vi "APXTurboEPICS.vi"() -> ()   [LabVIEW 2015]
uses:
  <vilib>/Instr/_visa.llb/VISA Configure Serial Port (Instr).vi
  <userlib>/caLab/Private/Get_PV-1D.vi
  <userlib>/caLab/Private/Put_DBL_PV.vi
  <userlib>/caLab/Private/Put_DBL-1D_PV-1D.vi
panel:
  out "APX:GASTurbo_START":bool
  out "APX:GASTrubo_STOP":bool
  out "APX:GASTurboF":dbl caption="F_20/Hz"
  out "APX:GASTurboP":dbl caption="P_20/W"
  out "APX:GASTurboS:STR":string
  out "APX:GASTurboS":dbl
  out "SERIAL 5":string
  out "GASTurbo":refnum<visa-resource-name>="COM4"
  out "APX:HPCTurbo_START":bool
  out "APX:HPCTrubo_STOP":bool
  out "APX:HPCTurboF":dbl caption="F_20/Hz"
  out "APX:HPCTurboP":dbl caption="P_20/W"
  out "APX:HPCTurboS:STR":string
  out "APX:HPCTurboS":dbl
  out "SERIAL 4":string
  out "HPCTurbo":refnum<visa-resource-name>="COM4"
  out "SERIAL 3":string
  out "L2Turbo":refnum<visa-resource-name>="COM4"
  out "APX:L2Turbo_START":bool
  out "APX:L2Turbo_STOP":bool
  out "APX:L2TurboF":dbl caption="F_20/Hz"
  out "APX:L2TurboP":dbl caption="P_20/W"
  out "APX:L2TurboS:STR":string
  out "AP2:L2TruboS":dbl
  out "SERIAL 2":string
  out "AP2Turbo":refnum<visa-resource-name>="COM4"
  out "APX:AP2Turbo_START":bool
  out "APX:AP2Trubo_STOP":bool
  out "APX:AP2TurboF":dbl caption="F_20/Hz"
  out "APX:AP2TurboP":dbl caption="P_20/W"
  out "APX:AP2TurboS:STR":string
  out "APX:AP2TruboS":dbl
  out "APX:HEMTurboS":dbl
  out "APX:HEMTurbo_STOP":bool
  out "APX:HEMTurbo_START":bool
  out "HEMTurbo":refnum<visa-resource-name>="COM4"
  out "APX:HEMTurboF":dbl caption="F_20/Hz"
  out "APX:HEMTurboP":dbl caption="P_20/W"
  out "APX:HEMTurboS:STR":string
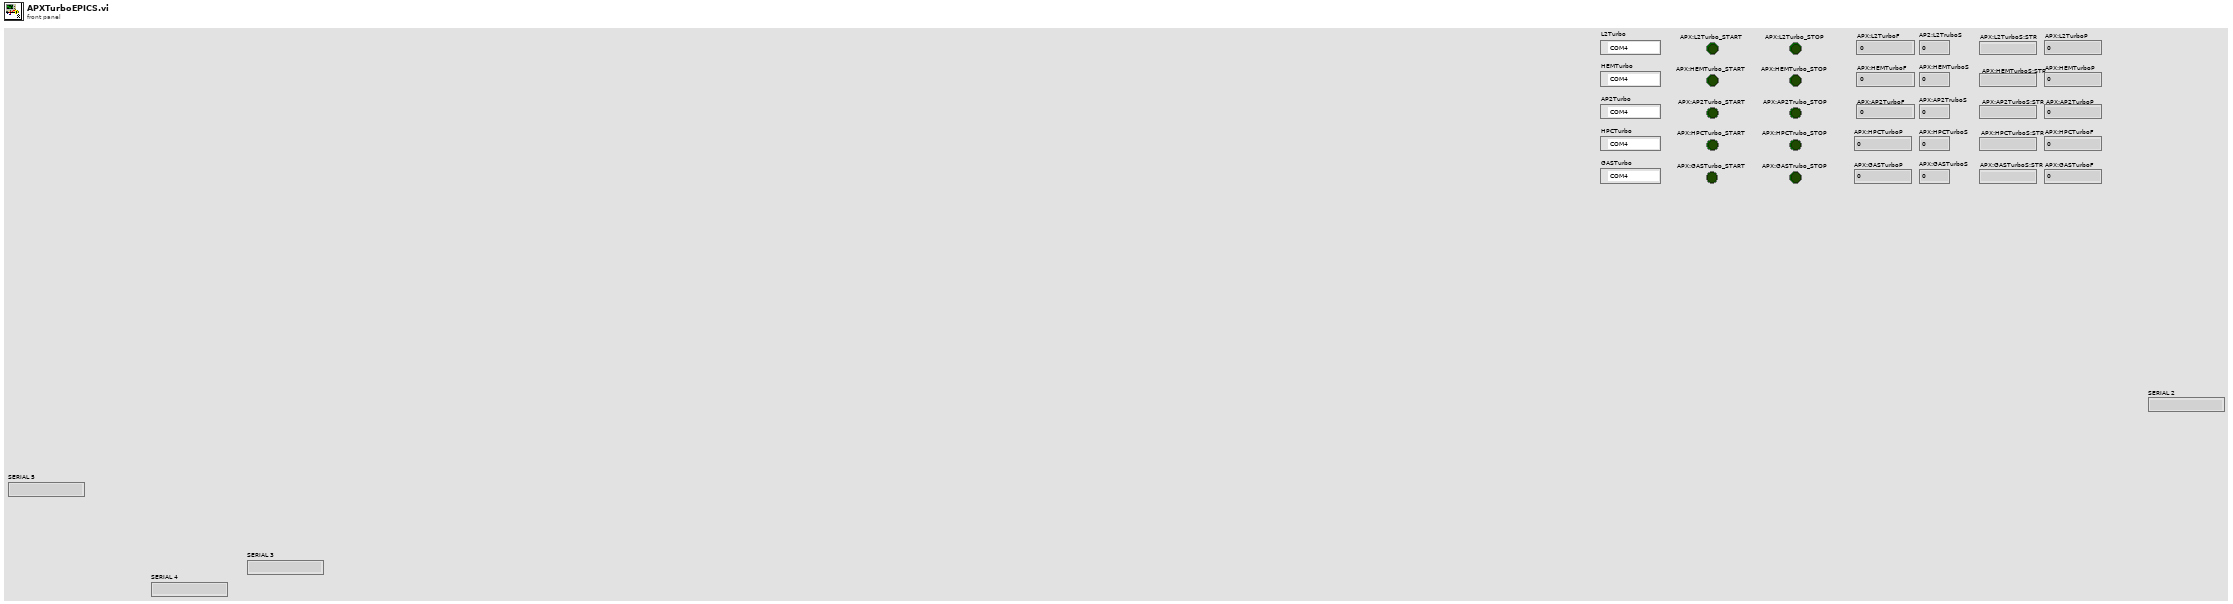
[diagram p1: front panel]
types:
  T1 = enum16{"START", "STOP", "REMOTE/SERIAL", "REMOTE", "SERIAL", "START/STOP", "PUMP STATUS", "Driving Frequency", "PUMP POWER", "PRESSURE"}
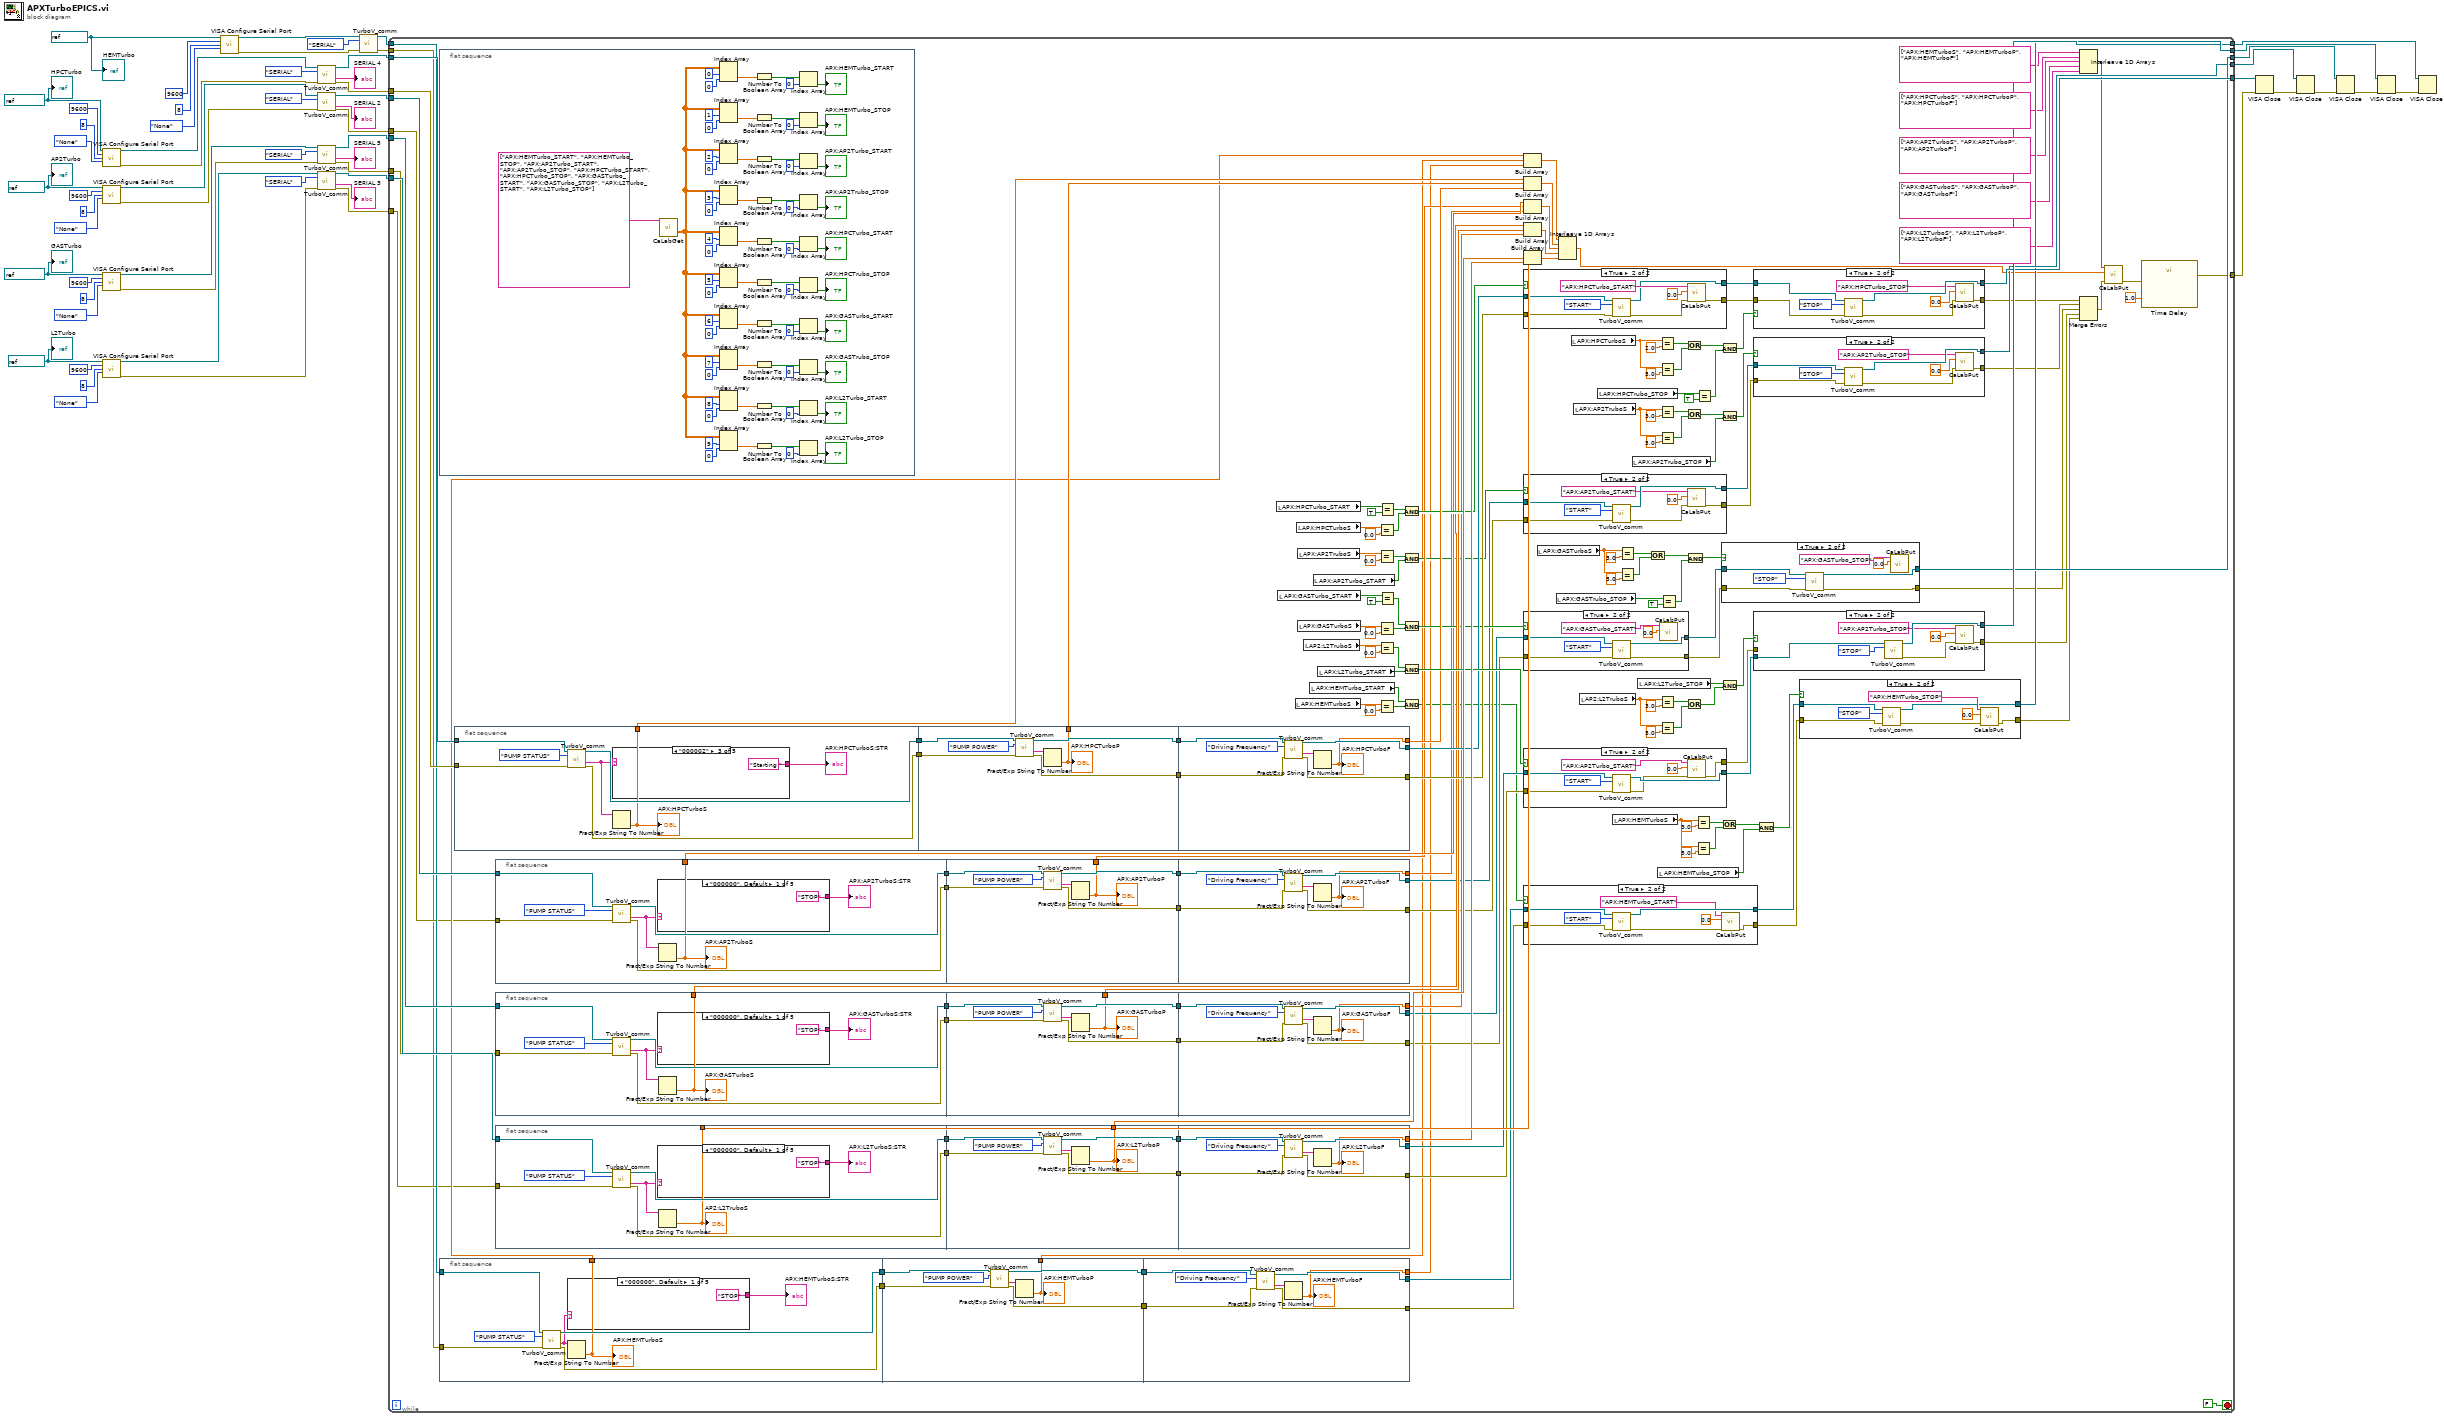
[diagram p0: block diagram]
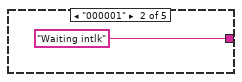
[diagram p2: hidden frame]
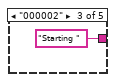
[diagram p3: hidden frame]
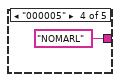
[diagram p4: hidden frame]
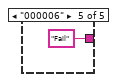
[diagram p5: hidden frame]
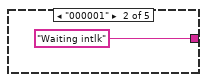
[diagram p8: hidden frame]
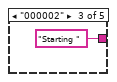
[diagram p9: hidden frame]
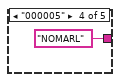
[diagram p10: hidden frame]
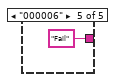
[diagram p11: hidden frame]
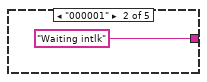
[diagram p14: hidden frame]
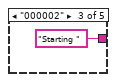
[diagram p15: hidden frame]
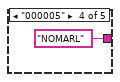
[diagram p16: hidden frame]
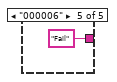
[diagram p17: hidden frame]
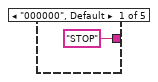
[diagram p20: hidden frame]
diagram:
  w18 = refnum<visa-resource-name> "COM25" ("VISA resource name")
  w33 = refnum<visa-resource-name> "COM26" ("VISA resource name")
  w44 = refnum<visa-resource-name> "COM4" ("VISA resource name")
  w52 = refnum<visa-resource-name> "COM6" ("VISA resource name")
  w59 = refnum<visa-resource-name> "COM5" ("VISA resource name")
  n1 = call-poly "VISA Configure Serial Port"("VISA resource name"=w18, "baud rate (9600)"=u32 9600, "data bits (8)"=u16 8, "parity (0:none)"=enum16{"None", "Odd", "Even", "Mark", "Space"}."None") -> ("VISA resource name out"=w23:refnum<visa-resource-name>, "error out"=w24:errorcluster)  [unwired: 10 in]
  n2 = call-poly "VISA Configure Serial Port"("VISA resource name"=w52, "baud rate (9600)"=u32 9600, "data bits (8)"=u16 8, "parity (0:none)"=enum16{"None", "Odd", "Even", "Mark", "Space"}."None") -> ("VISA resource name out"=w47:refnum<visa-resource-name>, "error out"=w46:errorcluster)  [unwired: 10 in]
  n3 = call-poly "VISA Configure Serial Port"("VISA resource name"=w33, "baud rate (9600)"=u32 9600, "data bits (8)"=u16 8, "parity (0:none)"=enum16{"None", "Odd", "Even", "Mark", "Space"}."None") -> ("VISA resource name out"=w28:refnum<visa-resource-name>, "error out"=w27:errorcluster)  [unwired: 10 in]
  n4 = call-poly "VISA Configure Serial Port"("VISA resource name"=w44, "baud rate (9600)"=u32 9600, "data bits (8)"=u16 8, "parity (0:none)"=enum16{"None", "Odd", "Even", "Mark", "Space"}."None") -> ("VISA resource name out"=w38:refnum<visa-resource-name>, "error out"=w36:errorcluster)  [unwired: 10 in]
  n5 = call-poly "VISA Configure Serial Port"("VISA resource name"=w59, "baud rate (9600)"=u32 9600, "data bits (8)"=u16 8, "parity (0:none)"=enum16{"None", "Odd", "Even", "Mark", "Space"}."None") -> ("VISA resource name out"=w54:refnum<visa-resource-name>, "error out"=w53:errorcluster)  [unwired: 10 in]
  n6 = call "TurboV_comm.vi"("VISA resource name"=w23, "Command"=T1."SERIAL", "error in (no error)"=w24) -> ("VISA resource name out"=w17:refnum<visa-resource-name>, "read buffer"=→"SERIAL 4":string, "error out"=w16:errorcluster)  [unwired: 10 in]
  n7 = call "TurboV_comm.vi"("VISA resource name"=w47, "Command"=T1."SERIAL", "error in (no error)"=w46) -> ("VISA resource name out"=w10:refnum<visa-resource-name>, "read buffer"=→"SERIAL 2":string, "error out"=w9:errorcluster)  [unwired: 10 in]
  n8 = call "TurboV_comm.vi"("VISA resource name"=w28, "Command"=T1."SERIAL", "error in (no error)"=w27) -> ("VISA resource name out"=w13:refnum<visa-resource-name>, "read buffer"=→"SERIAL 5":string, "error out"=w12:errorcluster)  [unwired: 10 in]
  n9 = call "TurboV_comm.vi"("VISA resource name"=w38, "Command"=T1."SERIAL", "error in (no error)"=w36) -> ("VISA resource name out"=w37:refnum<visa-resource-name>, "read buffer"=→"SERIAL 3":string, "error out"=w35:errorcluster)  [unwired: 10 in]
  n10 = call "TurboV_comm.vi"("VISA resource name"=w54, "Command"=T1."SERIAL", "error in (no error)"=w53) -> ("VISA resource name out"=w7:refnum<visa-resource-name>, "error out"=w6:errorcluster)  [unwired: 10 in, 1 out]
  n11 = while {
    tunnel: w37 -> [w224]
    tunnel: w35 -> [w82]
    tunnel: [w204] -> w40
    tunnel: w17 -> [w197]
    tunnel: w16 -> [w196]
    tunnel: [w167] -> w15
    tunnel: [w79] -> w14
    tunnel: w13 -> [w166]
    tunnel: w12 -> [w165]
    tunnel: [w164] -> w11
    tunnel: w10 -> [w135]
    tunnel: w9 -> [w83]
    tunnel: [w110] -> w8
    tunnel: w7 -> [w109]
    tunnel: w6 -> [w81]
    tunnel: [w80] -> w2
    stop <- FALSE stop-if-true
    n12 = flat-sequence {
      frame #0 {
        n13 = call-poly "CaLabGet.vi"("PV Names"=string[] ["APX:HEMTurbo_START", "APX:HEMTurbo_STOP", "APX:AP2Turbo_START", "APX:AP2Turbo_STOP", "APX:HPCTurbo_START", "APX:HPCTurbo_STOP", "APX:GASTurbo_START", "APX:GASTurbo_STOP", "APX:L2Turbo_START", "APX:L2Turbo_STOP"]) -> ("Value Array (number)"=w225:dbl[][])  [unwired: 8 in, 6 out]
        n14 = Index Array(array=w225, index (row)=0 ("disabled index (row)"), index (col)=0 ("index (row)")) -> (element=w233:dbl)
        n15 = Index Array(array=w225, index (row)=1 ("disabled index (row)"), index (col)=0 ("index (row)")) -> (element=w228:dbl)
        n16 = Index Array(array=w225, index (row)=2 ("disabled index (row)"), index (col)=0 ("index (row)")) -> (element=w246:dbl)
        n17 = Index Array(array=w225, index (row)=3 ("disabled index (row)"), index (col)=0 ("index (row)")) -> (element=w241:dbl)
        n18 = Index Array(array=w225, index (row)=4 ("disabled index (row)"), index (col)=0 ("index (row)")) -> (element=w270:dbl)
        n19 = Index Array(array=w225, index (row)=5 ("disabled index (row)"), index (col)=0 ("index (row)")) -> (element=w264:dbl)
        n20 = Index Array(array=w225, index (row)=6 ("disabled index (row)"), index (col)=0 ("index (row)")) -> (element=w258:dbl)
        n21 = Index Array(array=w225, index (row)=7 ("disabled index (row)"), index (col)=0 ("index (row)")) -> (element=w253:dbl)
        n22 = Index Array(array=w225, index (row)=8 ("disabled index (row)"), index (col)=0 ("index (row)")) -> (element=w282:dbl)
        n23 = Index Array(array=w225, index (row)=9 ("disabled index (row)"), index (col)=0 ("index (row)")) -> (element=w277:dbl)
        n24 = Number To Boolean Array(number=w233) -> (Boolean array=w235:bool[])
        n25 = Number To Boolean Array(number=w228) -> (Boolean array=w230:bool[])
        n26 = Number To Boolean Array(number=w246) -> (Boolean array=w248:bool[])
        n27 = Number To Boolean Array(number=w241) -> (Boolean array=w243:bool[])
        n28 = Number To Boolean Array(number=w270) -> (Boolean array=w272:bool[])
        n29 = Number To Boolean Array(number=w264) -> (Boolean array=w266:bool[])
        n30 = Number To Boolean Array(number=w258) -> (Boolean array=w260:bool[])
        n31 = Number To Boolean Array(number=w253) -> (Boolean array=w255:bool[])
        n32 = Number To Boolean Array(number=w282) -> (Boolean array=w284:bool[])
        n33 = Number To Boolean Array(number=w277) -> (Boolean array=w279:bool[])
        n34 = Index Array(array=w235, index=0) -> (element=→"APX:HEMTurbo_START":bool)
        n35 = Index Array(array=w230, index=0) -> (element=→"APX:HEMTurbo_STOP":bool)
        n36 = Index Array(array=w248, index=0) -> (element=→"APX:AP2Turbo_START":bool)
        n37 = Index Array(array=w243, index=0) -> (element=→"APX:AP2Trubo_STOP":bool)
        n38 = Index Array(array=w272, index=0) -> (element=→"APX:HPCTurbo_START":bool)
        n39 = Index Array(array=w266, index=0) -> (element=→"APX:HPCTrubo_STOP":bool)
        n40 = Index Array(array=w260, index=0) -> (element=→"APX:GASTurbo_START":bool)
        n41 = Index Array(array=w255, index=0) -> (element=→"APX:GASTrubo_STOP":bool)
        n42 = Index Array(array=w284, index=0) -> (element=→"APX:L2Turbo_START":bool)
        n43 = Index Array(array=w279, index=0) -> (element=→"APX:L2Turbo_STOP":bool)
      }
    }
    n44 = flat-sequence {
      tunnel: w109 -> [w294]
      tunnel: w81 -> [w293]
      tunnel: [w292] -> w107
      tunnel: [w291] -> w106
      tunnel: [w287] -> w103
      tunnel: w107 -> [w305]
      tunnel: w106 -> [w302]
      tunnel: [w304] -> w105
      tunnel: [w303] -> w104
      tunnel: [w300] -> w102
      tunnel: w105 -> [w313]
      tunnel: w104 -> [w312]
      tunnel: [w309] -> w92
      tunnel: [w308] -> w108
      tunnel: [w307] -> w101
      frame #0 {
        n45 = call "TurboV_comm.vi"("VISA resource name"=w294, "Command"=T1."PUMP STATUS", "error in (no error)"=w293) -> ("VISA resource name out"=w292:refnum<visa-resource-name>, "read buffer"=w288:string, "error out"=w291:errorcluster)  [unwired: 10 in]
        n46 = case shown="\"000000\", Default" w288 {
          tunnel: ["STOP" "Waiting intlk" "Starting " "NOMARL" "Fail"] -> w289
          frame "000000", Default {
          }
          frame "000001" {
          }
          frame "000002" {
          }
          frame "000005" {
          }
          frame "000006" {
          }
        }
        "APX:HEMTurboS:STR" <- w289
        n47 = Fract/Exp String To Number(string=w288) -> (number=w287:dbl)  [unwired: 3 in, 1 out]
        "APX:HEMTurboS" <- w287
      }
      frame #1 {
        n48 = call "TurboV_comm.vi"("VISA resource name"=w305, "Command"=T1."PUMP POWER", "error in (no error)"=w302) -> ("VISA resource name out"=w304:refnum<visa-resource-name>, "read buffer"=w301:string, "error out"=w303:errorcluster)  [unwired: 10 in]
        n49 = Fract/Exp String To Number(string=w301) -> (number=w300:dbl)  [unwired: 3 in, 1 out]
        "APX:HEMTurboP" <- w300
      }
      frame #2 {
        n50 = call "TurboV_comm.vi"("VISA resource name"=w313, "Command"=T1."Driving Frequency", "error in (no error)"=w312) -> ("VISA resource name out"=w308:refnum<visa-resource-name>, "read buffer"=w310:string, "error out"=w309:errorcluster)  [unwired: 10 in]
        n51 = Fract/Exp String To Number(string=w310) -> (number=w307:dbl)  [unwired: 3 in, 1 out]
        "APX:HEMTurboF" <- w307
      }
    }
    n52 = flat-sequence {
      tunnel: w197 -> [w433]
      tunnel: w196 -> [w432]
      tunnel: [w431] -> w195
      tunnel: [w430] -> w194
      tunnel: [w426] -> w191
      tunnel: w195 -> [w444]
      tunnel: w194 -> [w441]
      tunnel: [w443] -> w193
      tunnel: [w442] -> w192
      tunnel: [w439] -> w190
      tunnel: w193 -> [w452]
      tunnel: w192 -> [w451]
      tunnel: [w448] -> w179
      tunnel: [w447] -> w180
      tunnel: [w446] -> w189
      frame #0 {
        n53 = call "TurboV_comm.vi"("VISA resource name"=w433, "Command"=T1."PUMP STATUS", "error in (no error)"=w432) -> ("VISA resource name out"=w431:refnum<visa-resource-name>, "read buffer"=w427:string, "error out"=w430:errorcluster)  [unwired: 10 in]
        n54 = case shown="\"000002\"" w427 {
          tunnel: ["STOP" "Waiting intlk" "Starting " "NOMARL" "Fail"] -> w428
          frame "000000", Default {
          }
          frame "000001" {
          }
          frame "000002" {
          }
          frame "000005" {
          }
          frame "000006" {
          }
        }
        "APX:HPCTurboS:STR" <- w428
        n55 = Fract/Exp String To Number(string=w427) -> (number=w426:dbl)  [unwired: 3 in, 1 out]
        "APX:HPCTurboS" <- w426
      }
      frame #1 {
        n56 = call "TurboV_comm.vi"("VISA resource name"=w444, "Command"=T1."PUMP POWER", "error in (no error)"=w441) -> ("VISA resource name out"=w443:refnum<visa-resource-name>, "read buffer"=w440:string, "error out"=w442:errorcluster)  [unwired: 10 in]
        n57 = Fract/Exp String To Number(string=w440) -> (number=w439:dbl)  [unwired: 3 in, 1 out]
        "APX:HPCTurboP" <- w439
      }
      frame #2 {
        n58 = call "TurboV_comm.vi"("VISA resource name"=w452, "Command"=T1."Driving Frequency", "error in (no error)"=w451) -> ("VISA resource name out"=w447:refnum<visa-resource-name>, "read buffer"=w449:string, "error out"=w448:errorcluster)  [unwired: 10 in]
        n59 = Fract/Exp String To Number(string=w449) -> (number=w446:dbl)  [unwired: 3 in, 1 out]
        "APX:HPCTurboF" <- w446
      }
    }
    n60 = flat-sequence {
      tunnel: w135 -> [w341]
      tunnel: w83 -> [w340]
      tunnel: [w339] -> w134
      tunnel: [w338] -> w133
      tunnel: [w334] -> w130
      tunnel: w134 -> [w352]
      tunnel: w133 -> [w349]
      tunnel: [w351] -> w132
      tunnel: [w350] -> w131
      tunnel: [w347] -> w129
      tunnel: w132 -> [w360]
      tunnel: w131 -> [w359]
      tunnel: [w356] -> w120
      tunnel: [w355] -> w128
      tunnel: [w354] -> w119
      frame #0 {
        n61 = call "TurboV_comm.vi"("VISA resource name"=w341, "Command"=T1."PUMP STATUS", "error in (no error)"=w340) -> ("VISA resource name out"=w339:refnum<visa-resource-name>, "read buffer"=w335:string, "error out"=w338:errorcluster)  [unwired: 10 in]
        n62 = case shown="\"000000\", Default" w335 {
          tunnel: ["STOP" "Waiting intlk" "Starting " "NOMARL" "Fail"] -> w336
          frame "000000", Default {
          }
          frame "000001" {
          }
          frame "000002" {
          }
          frame "000005" {
          }
          frame "000006" {
          }
        }
        "APX:AP2TurboS:STR" <- w336
        n63 = Fract/Exp String To Number(string=w335) -> (number=w334:dbl)  [unwired: 3 in, 1 out]
        "APX:AP2TruboS" <- w334
      }
      frame #1 {
        n64 = call "TurboV_comm.vi"("VISA resource name"=w352, "Command"=T1."PUMP POWER", "error in (no error)"=w349) -> ("VISA resource name out"=w351:refnum<visa-resource-name>, "read buffer"=w348:string, "error out"=w350:errorcluster)  [unwired: 10 in]
        n65 = Fract/Exp String To Number(string=w348) -> (number=w347:dbl)  [unwired: 3 in, 1 out]
        "APX:AP2TurboP" <- w347
      }
      frame #2 {
        n66 = call "TurboV_comm.vi"("VISA resource name"=w360, "Command"=T1."Driving Frequency", "error in (no error)"=w359) -> ("VISA resource name out"=w356:refnum<visa-resource-name>, "read buffer"=w357:string, "error out"=w354:errorcluster)  [unwired: 10 in]
        n67 = Fract/Exp String To Number(string=w357) -> (number=w355:dbl)  [unwired: 3 in, 1 out]
        "APX:AP2TurboF" <- w355
      }
    }
    n68 = flat-sequence {
      tunnel: [w388] -> w163
      tunnel: [w387] -> w162
      tunnel: [w383] -> w159
      tunnel: w166 -> [w382]
      tunnel: w165 -> [w381]
      tunnel: w163 -> [w399]
      tunnel: w162 -> [w396]
      tunnel: [w398] -> w161
      tunnel: [w397] -> w160
      tunnel: [w394] -> w158
      tunnel: w161 -> [w407]
      tunnel: w160 -> [w406]
      tunnel: [w403] -> w136
      tunnel: [w402] -> w137
      tunnel: [w401] -> w157
      frame #0 {
        n69 = call "TurboV_comm.vi"("VISA resource name"=w382, "Command"=T1."PUMP STATUS", "error in (no error)"=w381) -> ("VISA resource name out"=w388:refnum<visa-resource-name>, "read buffer"=w384:string, "error out"=w387:errorcluster)  [unwired: 10 in]
        n70 = case shown="\"000000\", Default" w384 {
          tunnel: ["STOP" "Waiting intlk" "Starting " "NOMARL" "Fail"] -> w385
          frame "000000", Default {
          }
          frame "000001" {
          }
          frame "000002" {
          }
          frame "000005" {
          }
          frame "000006" {
          }
        }
        "APX:GASTurboS:STR" <- w385
        n71 = Fract/Exp String To Number(string=w384) -> (number=w383:dbl)  [unwired: 3 in, 1 out]
        "APX:GASTurboS" <- w383
      }
      frame #1 {
        n72 = call "TurboV_comm.vi"("VISA resource name"=w399, "Command"=T1."PUMP POWER", "error in (no error)"=w396) -> ("VISA resource name out"=w398:refnum<visa-resource-name>, "read buffer"=w395:string, "error out"=w397:errorcluster)  [unwired: 10 in]
        n73 = Fract/Exp String To Number(string=w395) -> (number=w394:dbl)  [unwired: 3 in, 1 out]
        "APX:GASTurboP" <- w394
      }
      frame #2 {
        n74 = call "TurboV_comm.vi"("VISA resource name"=w407, "Command"=T1."Driving Frequency", "error in (no error)"=w406) -> ("VISA resource name out"=w402:refnum<visa-resource-name>, "read buffer"=w404:string, "error out"=w403:errorcluster)  [unwired: 10 in]
        n75 = Fract/Exp String To Number(string=w404) -> (number=w401:dbl)  [unwired: 3 in, 1 out]
        "APX:GASTurboF" <- w401
      }
    }
    n76 = flat-sequence {
      tunnel: w224 -> [w480]
      tunnel: w82 -> [w479]
      tunnel: [w478] -> w212
      tunnel: [w477] -> w211
      tunnel: [w473] -> w222
      tunnel: w212 -> [w491]
      tunnel: w211 -> [w488]
      tunnel: [w490] -> w210
      tunnel: [w489] -> w209
      tunnel: [w486] -> w221
      tunnel: w210 -> [w499]
      tunnel: w209 -> [w498]
      tunnel: [w495] -> w207
      tunnel: [w494] -> w208
      tunnel: [w493] -> w220
      frame #0 {
        n77 = call "TurboV_comm.vi"("VISA resource name"=w480, "Command"=T1."PUMP STATUS", "error in (no error)"=w479) -> ("VISA resource name out"=w478:refnum<visa-resource-name>, "read buffer"=w474:string, "error out"=w477:errorcluster)  [unwired: 10 in]
        n78 = case shown="\"000000\", Default" w474 {
          tunnel: ["STOP" "Waiting intlk" "Starting " "NOMARL" "Fail"] -> w475
          frame "000000", Default {
          }
          frame "000001" {
          }
          frame "000002" {
          }
          frame "000005" {
          }
          frame "000006" {
          }
        }
        "APX:L2TurboS:STR" <- w475
        n79 = Fract/Exp String To Number(string=w474) -> (number=w473:dbl)  [unwired: 3 in, 1 out]
        "AP2:L2TruboS" <- w473
      }
      frame #1 {
        n80 = call "TurboV_comm.vi"("VISA resource name"=w491, "Command"=T1."PUMP POWER", "error in (no error)"=w488) -> ("VISA resource name out"=w490:refnum<visa-resource-name>, "read buffer"=w487:string, "error out"=w489:errorcluster)  [unwired: 10 in]
        n81 = Fract/Exp String To Number(string=w487) -> (number=w486:dbl)  [unwired: 3 in, 1 out]
        "APX:L2TurboP" <- w486
      }
      frame #2 {
        n82 = call "TurboV_comm.vi"("VISA resource name"=w499, "Command"=T1."Driving Frequency", "error in (no error)"=w498) -> ("VISA resource name out"=w494:refnum<visa-resource-name>, "read buffer"=w496:string, "error out"=w495:errorcluster)  [unwired: 10 in]
        n83 = Fract/Exp String To Number(string=w496) -> (number=w493:dbl)  [unwired: 3 in, 1 out]
        "APX:L2TurboF" <- w493
      }
    }
    n84 = local read "APX:HPCTurbo_START"() -> (w168:bool)
    n85 = local read "APX:GASTurbo_START"() -> (w154:bool)
    n86 = local read "APX:HEMTurboS"() -> (w94:dbl)
    n87 = local read "APX:HPCTurboS"() -> (w187:dbl)
    n88 = local read "APX:AP2TruboS"() -> (w121:dbl)
    n89 = local read "APX:GASTurboS"() -> (w155:dbl)
    n90 = local read "AP2:L2TruboS"() -> (w218:dbl)
    n91 = local read "APX:HEMTurbo_START"() -> (w89:bool)
    n92 = local read "APX:AP2Turbo_START"() -> (w114:bool)
    n93 = local read "APX:L2Turbo_START"() -> (w198:bool)
    n94 = Equal?(x=w187, y=0.0) -> (x = y?=w172:bool)
    n95 = Equal?(x=w121, y=0.0) -> (x = y?=w116:bool)
    n96 = Equal?(x=w155, y=0.0) -> (x = y?=w151:bool)
    n97 = Equal?(x=w218, y=0.0) -> (x = y?=w200:bool)
    n98 = Equal?(x=w94, y=0.0) -> (x = y?=w88:bool)
    n99 = Equal?(x=w168, y=TRUE) -> (x = y?=w170:bool)
    n100 = Equal?(x=w154, y=TRUE) -> (x = y?=w152:bool)
    n101 = And(x=w170, y=w172) -> (x .and. y?=w171:bool)
    n102 = And(x=w116, y=w114) -> (x .and. y?=w115:bool)
    n103 = And(x=w152, y=w151) -> (x .and. y?=w150:bool)
    n104 = And(x=w200, y=w198) -> (x .and. y?=w199:bool)
    n105 = And(x=w89, y=w88) -> (x .and. y?=w87:bool)
    n106 = Build Array(w103, w102, w101) -> (w73:dbl[])
    n107 = Build Array(w191, w190, w189) -> (w72:dbl[])
    n108 = Build Array(w130, w129, w128) -> (w64:dbl[])
    n109 = Build Array(w159, w158, w157) -> (w63:dbl[])
    n110 = Build Array(w222, w221, w220) -> (w62:dbl[])
    n111 = case shown="True" w171 {
      tunnel: [w464 w466] -> w177
      tunnel: w180 -> [w463 w471]
      tunnel: w179 -> [w464 w470]
      tunnel: [w463 w465] -> w178
      frame False {
      }
      frame True {
        n112 = call "TurboV_comm.vi"("VISA resource name"=w471, "Command"=T1."START", "error in (no error)"=w470) -> ("VISA resource name out"=w465:refnum<visa-resource-name>, "error out"=w467:errorcluster)  [unwired: 10 in, 1 out]
        n113 = call-poly <userlib>:"CaLabPut.vi"("Error in (no error)"=w467, "Value"=0.0, "PV Name"="APX:HPCTurbo_START") -> ("Error out"=w466:errorcluster)  [unwired: 5 in, 3 out]
      }
    }
    n114 = case shown="True" w115 {
      tunnel: [w362 w369] -> w118
      tunnel: [w361 w363] -> w117
      tunnel: w120 -> [w362 w368]
      tunnel: w119 -> [w361 w367]
      frame False {
      }
      frame True {
        n115 = call "TurboV_comm.vi"("VISA resource name"=w368, "Command"=T1."START", "error in (no error)"=w367) -> ("VISA resource name out"=w369:refnum<visa-resource-name>, "error out"=w364:errorcluster)  [unwired: 10 in, 1 out]
        n116 = call-poly <userlib>:"CaLabPut.vi"("Error in (no error)"=w364, "Value"=0.0, "PV Name"="APX:AP2Turbo_START") -> ("Error out"=w363:errorcluster)  [unwired: 5 in, 3 out]
      }
    }
    n117 = case shown="True" w150 {
      tunnel: [w418 w424] -> w144
      tunnel: [w417 w423] -> w143
      tunnel: w137 -> [w418 w422]
      tunnel: w136 -> [w417 w421]
      frame False {
      }
      frame True {
        n118 = call "TurboV_comm.vi"("VISA resource name"=w422, "Command"=T1."START", "error in (no error)"=w421) -> ("VISA resource name out"=w424:refnum<visa-resource-name>, "error out"=w423:errorcluster)  [unwired: 10 in, 1 out]
        n119 = call-poly <userlib>:"CaLabPut.vi"("Value"=0.0, "PV Name"="APX:GASTurbo_START") -> ()  [unwired: 6 in, 4 out]
      }
    }
    n120 = case shown="True" w199 {
      tunnel: [w510 w517] -> w206
      tunnel: [w509 w511] -> w205
      tunnel: w208 -> [w510 w516]
      tunnel: w207 -> [w509 w515]
      frame False {
      }
      frame True {
        n121 = call "TurboV_comm.vi"("VISA resource name"=w516, "Command"=T1."START", "error in (no error)"=w515) -> ("VISA resource name out"=w517:refnum<visa-resource-name>, "error out"=w512:errorcluster)  [unwired: 10 in, 1 out]
        n122 = call-poly <userlib>:"CaLabPut.vi"("Error in (no error)"=w512, "Value"=0.0, "PV Name"="APX:AP2Turbo_START") -> ("Error out"=w511:errorcluster)  [unwired: 5 in, 3 out]
      }
    }
    n123 = case shown="True" w87 {
      tunnel: [w315 w322] -> w91
      tunnel: [w314 w316] -> w90
      tunnel: w108 -> [w315 w321]
      tunnel: w92 -> [w314 w320]
      frame False {
      }
      frame True {
        n124 = call "TurboV_comm.vi"("VISA resource name"=w321, "Command"=T1."START", "error in (no error)"=w320) -> ("VISA resource name out"=w322:refnum<visa-resource-name>, "error out"=w317:errorcluster)  [unwired: 10 in, 1 out]
        n125 = call-poly <userlib>:"CaLabPut.vi"("Error in (no error)"=w317, "Value"=0.0, "PV Name"="APX:HEMTurbo_START") -> ("Error out"=w316:errorcluster)  [unwired: 5 in, 3 out]
      }
    }
    n126 = local read "APX:GASTurboS"() -> (w145:dbl)
    n127 = local read "APX:GASTrubo_STOP"() -> (w139:bool)
    n128 = Interleave 1D Arrays(w73, w72, w64, w63, w62) -> (w71:dbl[])
    n129 = local read "APX:HPCTurboS"() -> (w183:dbl)
    n130 = local read "APX:AP2TruboS"() -> (w127:dbl)
    n131 = local read "AP2:L2TruboS"() -> (w217:dbl)
    n132 = local read "APX:HPCTrubo_STOP"() -> (w174:bool)
    n133 = local read "APX:HEMTurboS"() -> (w100:dbl)
    n134 = Equal?(x=w145, y=3.0) -> (x = y?=w147:bool)
    n135 = Equal?(x=w145, y=5.0) -> (x = y?=w146:bool)
    n136 = local read "APX:AP2Trubo_STOP"() -> (w111:bool)
    n137 = local read "APX:L2Turbo_STOP"() -> (w203:bool)
    n138 = Or(x=w147, y=w146) -> (x .or. y?=w141:bool)
    n139 = local read "APX:HEMTurbo_STOP"() -> (w84:bool)
    n140 = Equal?(x=w183, y=2.0) -> (x = y?=w184:bool)
    n141 = Equal?(x=w183, y=5.0) -> (x = y?=w185:bool)
    n142 = Equal?(x=w127, y=3.0) -> (x = y?=w125:bool)
    n143 = Equal?(x=w127, y=5.0) -> (x = y?=w126:bool)
    n144 = Equal?(x=w217, y=3.0) -> (x = y?=w215:bool)
    n145 = Equal?(x=w217, y=5.0) -> (x = y?=w216:bool)
    n146 = Equal?(x=w139, y=TRUE) -> (x = y?=w140:bool)
    n147 = Or(x=w184, y=w185) -> (x .or. y?=w186:bool)
    n148 = Or(x=w125, y=w126) -> (x .or. y?=w113:bool)
    n149 = Or(x=w215, y=w216) -> (x .or. y?=w202:bool)
    n150 = And(x=w141, y=w140) -> (x .and. y?=w142:bool)
    n151 = Equal?(x=w100, y=3.0) -> (x = y?=w98:bool)
    n152 = Equal?(x=w100, y=5.0) -> (x = y?=w99:bool)
    n153 = Equal?(x=w174, y=TRUE) -> (x = y?=w175:bool)
    n154 = Or(x=w98, y=w99) -> (x .or. y?=w86:bool)
    n155 = And(x=w186, y=w175) -> (x .and. y?=w176:bool)
    n156 = And(x=w113, y=w111) -> (x .and. y?=w112:bool)
    n157 = And(x=w203, y=w202) -> (x .and. y?=w201:bool)
    n158 = case shown="True" w142 {
      tunnel: [w409 w416] -> w164
      tunnel: [w408 w415] -> w76
      tunnel: w144 -> [w409 w413]
      tunnel: w143 -> [w408 w412]
      frame False {
      }
      frame True {
        n159 = call "TurboV_comm.vi"("VISA resource name"=w413, "Command"=T1."STOP", "error in (no error)"=w412) -> ("VISA resource name out"=w416:refnum<visa-resource-name>, "error out"=w415:errorcluster)  [unwired: 10 in, 1 out]
        n160 = call-poly <userlib>:"CaLabPut.vi"("Value"=0.0, "PV Name"="APX:GASTurbo_STOP") -> ()  [unwired: 6 in, 4 out]
      }
    }
    n161 = case shown="True" w176 {
      tunnel: [w454 w462] -> w167
      tunnel: [w453 w455] -> w78
      tunnel: w178 -> [w454 w461]
      tunnel: w177 -> [w453 w460]
      frame False {
      }
      frame True {
        n162 = call "TurboV_comm.vi"("VISA resource name"=w461, "Command"=T1."STOP", "error in (no error)"=w460) -> ("VISA resource name out"=w462:refnum<visa-resource-name>, "error out"=w456:errorcluster)  [unwired: 10 in, 1 out]
        n163 = call-poly <userlib>:"CaLabPut.vi"("Error in (no error)"=w456, "Value"=0.0, "PV Name"="APX:HPCTurbo_STOP") -> ("Error out"=w455:errorcluster)  [unwired: 5 in, 3 out]
      }
    }
    n164 = case shown="True" w112 {
      tunnel: [w372 w380] -> w110
      tunnel: [w371 w373] -> w77
      tunnel: w118 -> [w372 w379]
      tunnel: w117 -> [w371 w378]
      frame False {
      }
      frame True {
        n165 = call "TurboV_comm.vi"("VISA resource name"=w379, "Command"=T1."STOP", "error in (no error)"=w378) -> ("VISA resource name out"=w380:refnum<visa-resource-name>, "error out"=w374:errorcluster)  [unwired: 10 in, 1 out]
        n166 = call-poly <userlib>:"CaLabPut.vi"("Error in (no error)"=w374, "Value"=0.0, "PV Name"="APX:AP2Turbo_STOP") -> ("Error out"=w373:errorcluster)  [unwired: 5 in, 3 out]
      }
    }
    n167 = case shown="True" w201 {
      tunnel: [w501 w508] -> w204
      tunnel: [w500 w502] -> w75
      tunnel: w206 -> [w501 w507]
      tunnel: w205 -> [w500 _]
      frame False {
      }
      frame True {
        n168 = call "TurboV_comm.vi"("VISA resource name"=w507, "Command"=T1."STOP") -> ("VISA resource name out"=w508:refnum<visa-resource-name>, "error out"=w503:errorcluster)  [unwired: 11 in, 1 out]
        n169 = call-poly <userlib>:"CaLabPut.vi"("Error in (no error)"=w503, "Value"=0.0, "PV Name"="APX:AP2Turbo_STOP") -> ("Error out"=w502:errorcluster)  [unwired: 5 in, 3 out]
      }
    }
    n170 = And(x=w86, y=w84) -> (x .and. y?=w85:bool)
    n171 = case shown="True" w85 {
      tunnel: w91 -> [w325 w333]
      tunnel: w90 -> [w324 w332]
      tunnel: [w325 w328] -> w80
      tunnel: [w324 w326] -> w74
      frame False {
      }
      frame True {
        n172 = call "TurboV_comm.vi"("VISA resource name"=w333, "Command"=T1."STOP", "error in (no error)"=w332) -> ("VISA resource name out"=w328:refnum<visa-resource-name>, "error out"=w327:errorcluster)  [unwired: 10 in, 1 out]
        n173 = call-poly <userlib>:"CaLabPut.vi"("Error in (no error)"=w327, "Value"=0.0, "PV Name"="APX:HEMTurbo_STOP") -> ("Error out"=w326:errorcluster)  [unwired: 5 in, 3 out]
      }
    }
    n174 = Interleave 1D Arrays(string[] ["APX:HEMTurboS", "APX:HEMTurboP", "APX:HEMTurboF"], string[] ["APX:HPCTurboS", "APX:HPCTurboP", "APX:HPCTurboF"], string[] ["APX:AP2TurboS", "APX:AP2TurboP", "APX:AP2TurboF"], string[] ["APX:GASTurboS", "APX:GASTurboP", "APX:GASTurboF"], string[] ["APX:L2TurboS", "APX:L2TurboP", "APX:L2TurboF"]) -> (w65:string[])
    n175 = Merge Errors(w78, w77, w76, w75, w74) -> (w61:errorcluster)
    n176 = call-poly <userlib>:"CaLabPut.vi"("Error in (no error)"=w61, "Values"=w71, "PV Names"=w65) -> ("Error out"=w60:errorcluster)  [unwired: 5 in, 3 out]
    n177 = call "Time Delay"("error in (no error)"=w60, "Delay Time (s)"=1.0) -> ("error out"=w79:errorcluster)  [unwired: 9 in]
  }
  n178 = VISA Close(VISA resource name=w15, error in (no error)=w14) -> (error out=w5:errorcluster)
  n179 = VISA Close(VISA resource name=w8, error in (no error)=w5) -> (error out=w4:errorcluster)
  n180 = VISA Close(VISA resource name=w11, error in (no error)=w4) -> (error out=w3:errorcluster)
  n181 = VISA Close(VISA resource name=w40, error in (no error)=w3) -> (error out=w1:errorcluster)
  n182 = VISA Close(VISA resource name=w2, error in (no error)=w1) -> ()  [unwired: 1 out]
  "HEMTurbo" <- w59
  "AP2Turbo" <- w52
  "L2Turbo" <- w44
  "GASTurbo" <- w33
  "HPCTurbo" <- w18
